vi "Hide Module.vi"() -> ()   [LabVIEW 2014, in "Chart Module.lvlib"]
doc: "Hide the UI Front Panel of the module"
uses:
  Chart Module.lvlib
  Hide Panel Argument--cluster.ctl
panel:
  out "error out":errorcluster
  in  "error in":errorcluster
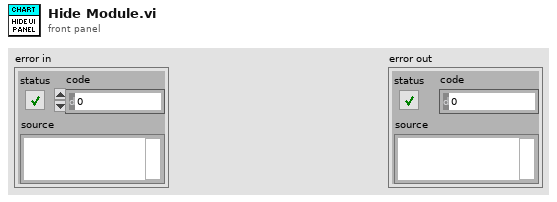
[diagram p1: front panel]
types:
  T1 = typedef "Chart Module.lvlib/Hide Panel Argument--cluster.ctl" = cluster{"Hide Panel?":bool}
  T2 = typedef "Chart Module.lvlib/Request Events--cluster.ctl" = cluster{"Stop Module":refnum<user-event>, "Show Panel":refnum<user-event>, "Hide Panel":refnum<user-event>}
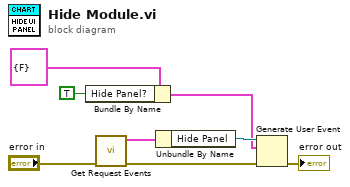
[diagram p0: block diagram]
diagram:
  n1 = Bundle By Name(cluster=T1 {"Hide Panel?"=FALSE} ("event data"), "Hide Panel?"=TRUE) -> (w4:T1)
  n2 = call "Get Request Events.vi"("error in"="error in") -> ("error out"=w3:errorcluster, "Request Events"=w8:T2)  [unwired: 9 in]
  n3 = Unbundle By Name(w8) -> ("Hide Panel"=w7:refnum<user-event>)
  n4 = Generate User Event(user event=w7, event data cluster=w4, error in=w3) -> (error out=→"error out":errorcluster)  [unwired: 1 in, 1 out]
